vi "Speed Loop.vi"(11 "FPGA Ref":T1) -> ()   [LabVIEW 2013]
uses:
  Controls/FPGA_Reference.ctl
  Type Defs/Pump Data Mode.ctl
  <vilib>/rvi/interface/common/niFpgaWaitOnOcc.vi
  <vilib>/Utility/error.llb/Error Cluster From Error Code.vi
  <vilib>/rvi/errors/niLvFpgaAdjustHostInterfaceError.vi
  <vilib>/rvi/interface/nirviMethod/nirviMethod.xnode
  FPGA/bitfiles/TI sbRIO PWM (FPGA) v1.0.lvbitx
  <vilib>/rvi/errors/niLvFpgaMergeErrorWithErrorCode.vi
  <vilib>/FPGAPlugInAG/sbRIO-9626/niLvFpga_ReadFifo_sbRIO-9626.vi
panel:
  in  "Boolean":bool
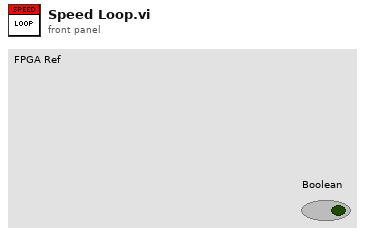
[diagram p1: front panel]
types:
  T1 = typedef "FPGA_Reference.ctl" = refnum<k20>
  T2 = cluster{"Calc 1":bool, "Calc 2":bool, "Calc 3":bool, "Calc 4":bool, "Calc 5":bool, "Calc 6":bool}
  T3 = cluster{"Array 1":dbl[], "Array 2":dbl[], "Array 3":dbl[], "Array 4":dbl[], "Array 5":dbl[], "Array 6":dbl[], "PreRead Pts":i32, "Calc Speed":cluster{"Calc 1":bool, "Calc 2":bool, "Calc 3":bool, "Calc 4":bool, "Calc 5":bool, "Calc 6":bool}, "LoopStartTime":dbl, "Speeds":dbl[], "Array 7":dbl[], "Array 8":dbl[], "Array 9":dbl[], "Array 10":dbl[], "Array 11":dbl[], "Array 12":dbl[], "Speeds 2":dbl[]}
  T4 = typedef "Pump Data Mode.ctl" = enum16{"Read", "Write Data", "Write Cal", "Write Watlow Data", "Write Pressure Offsets", "Write Initial Times", "Write Pumps Present", "Diagnostic Status", "Write Speed"}
  T5 = cluster{"max window":dbl, "min window":dbl, "CommSegments":dbl}
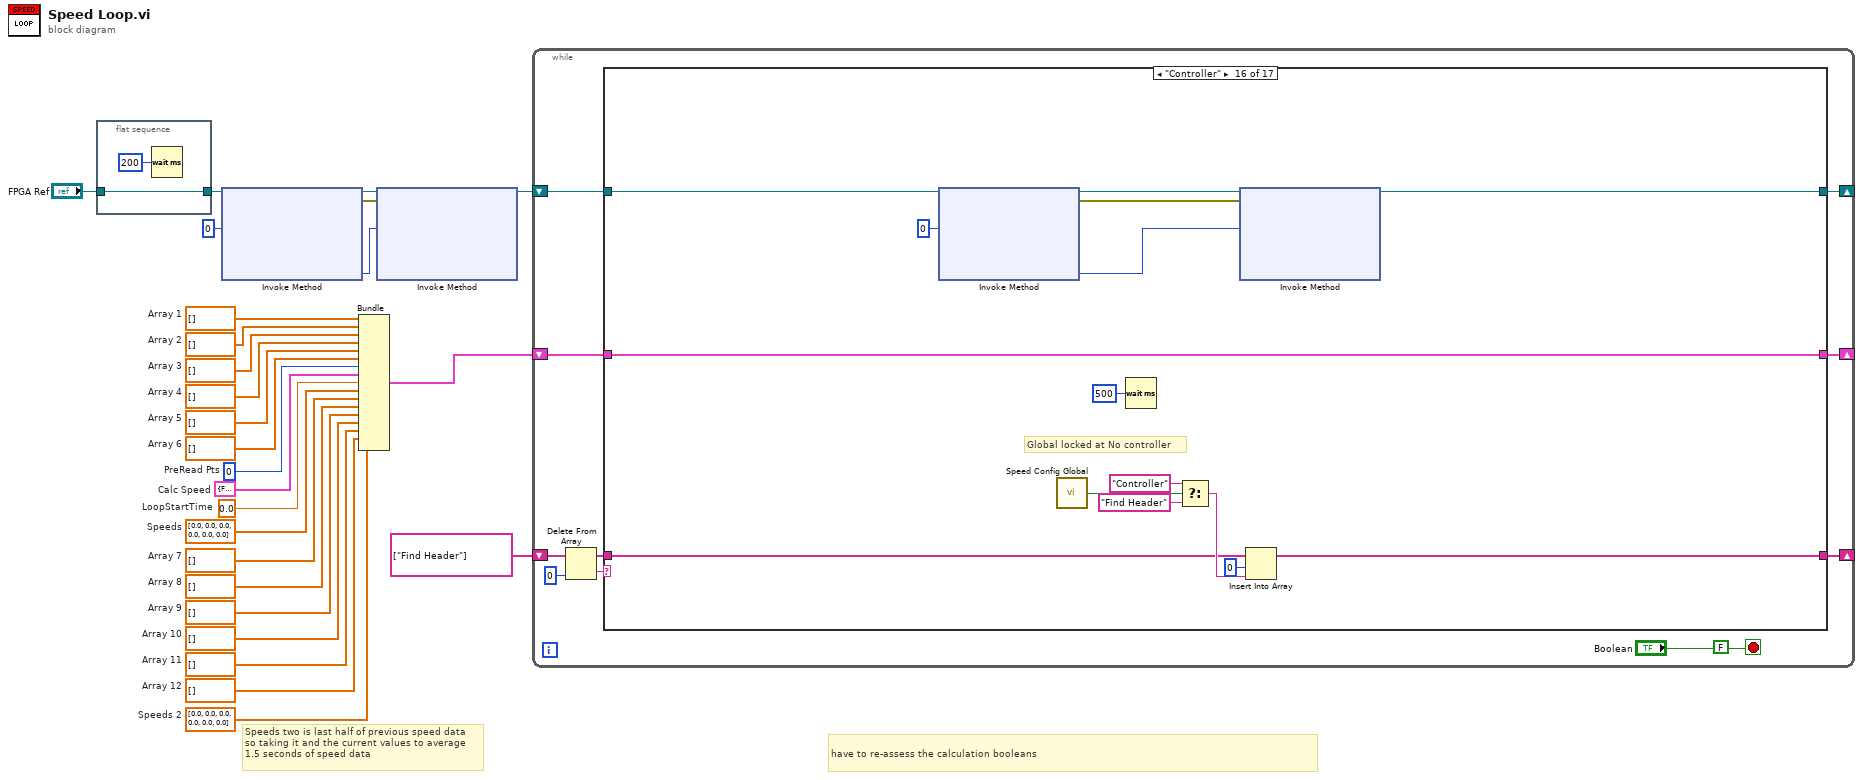
[diagram p0: block diagram]
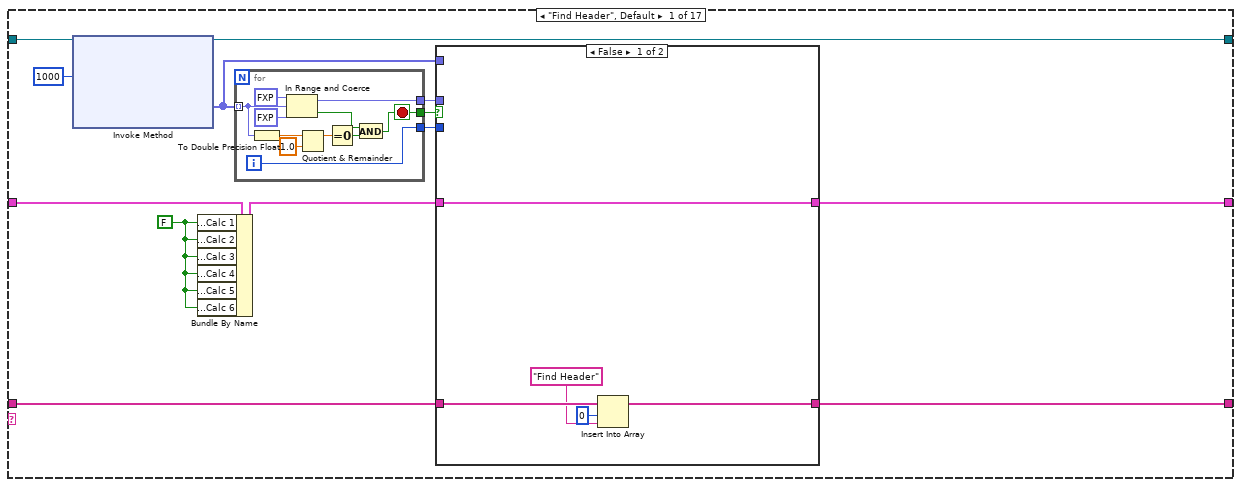
[diagram p2: hidden frame]
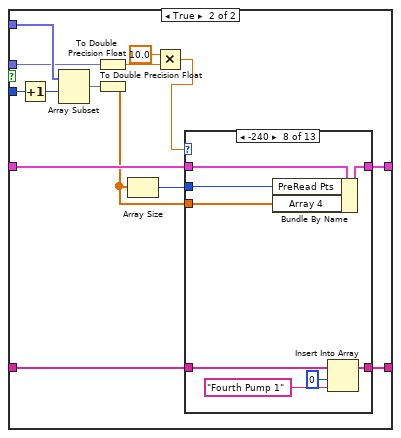
[diagram p3: hidden frame]
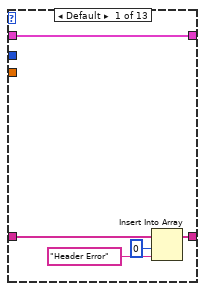
[diagram p4: hidden frame]
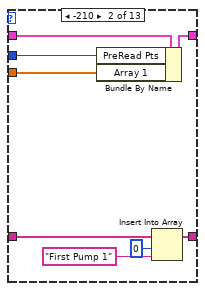
[diagram p5: hidden frame]
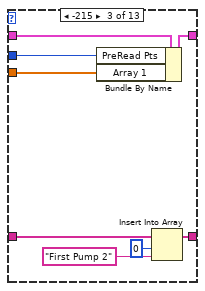
[diagram p6: hidden frame]
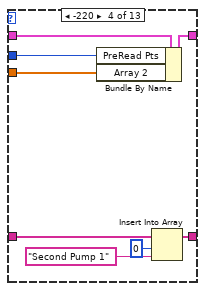
[diagram p7: hidden frame]
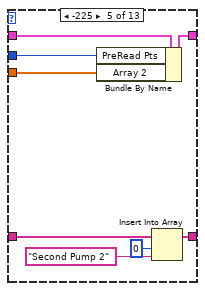
[diagram p8: hidden frame]
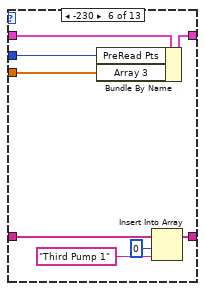
[diagram p9: hidden frame]
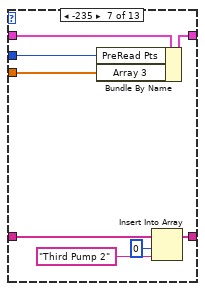
[diagram p10: hidden frame]
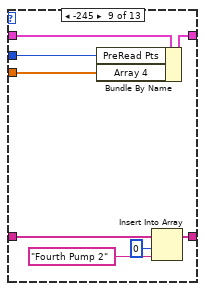
[diagram p11: hidden frame]
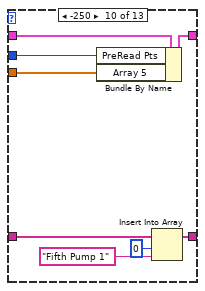
[diagram p12: hidden frame]
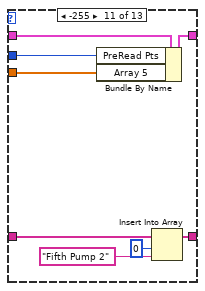
[diagram p13: hidden frame]
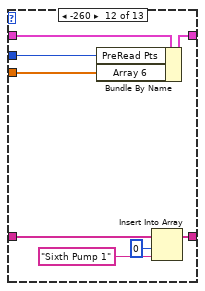
[diagram p14: hidden frame]
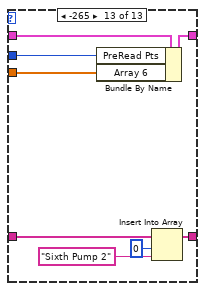
[diagram p15: hidden frame]
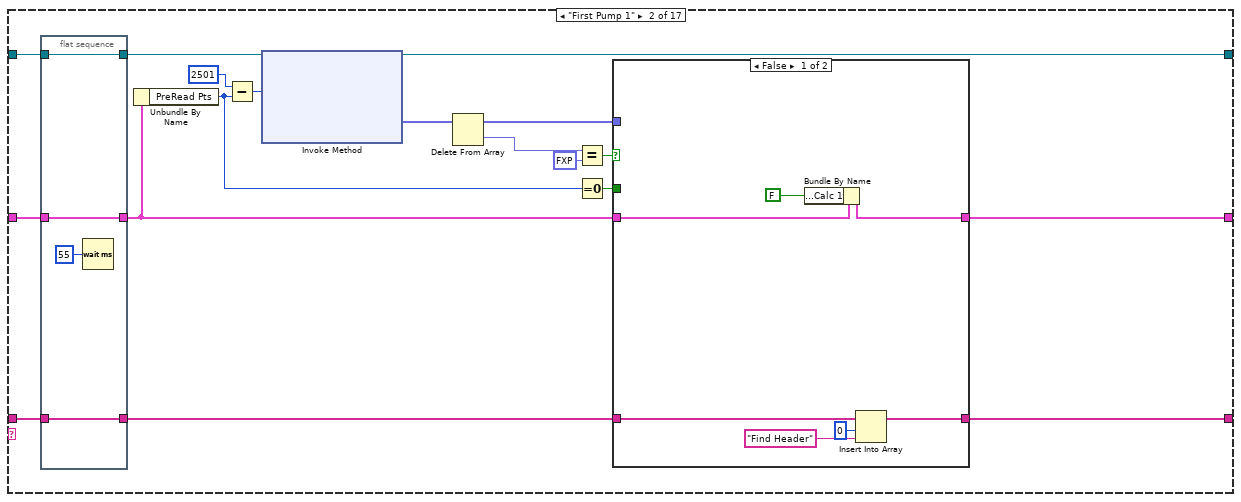
[diagram p16: hidden frame]
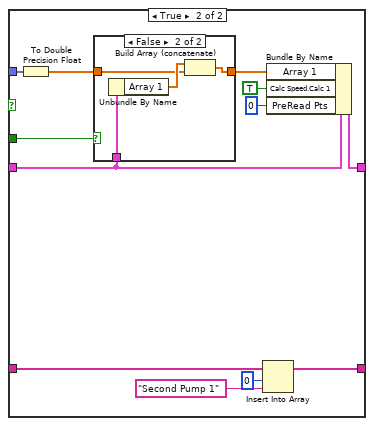
[diagram p17: hidden frame]
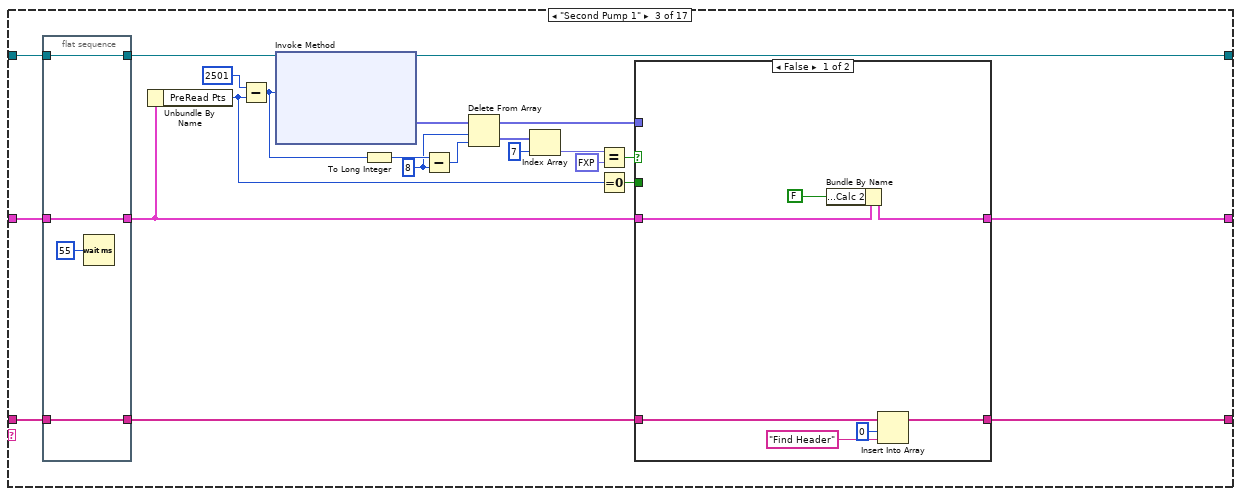
[diagram p19: hidden frame]
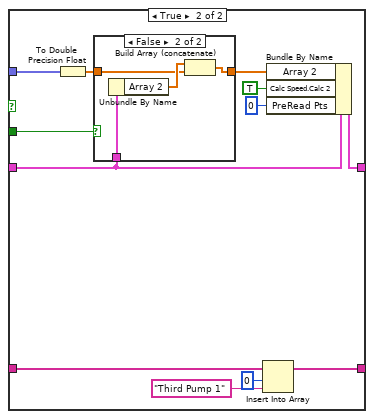
[diagram p20: hidden frame]
diagram:
  w1 = dbl[] [0.0, 0.0, 0.0, 0.0, 0.0, 0.0]  # Speeds 2
  w2 = dbl[] []  # Array 12
  w3 = dbl[] []  # Array 11
  w4 = dbl[] []  # Array 10
  w5 = dbl[] []  # Array 9
  w6 = dbl[] []  # Array 8
  w7 = dbl[] []  # Array 7
  w10 = dbl[] [0.0, 0.0, 0.0, 0.0, 0.0, 0.0]  # Speeds
  w11 = 0.0  # LoopStartTime
  w26 = T2 {"Calc 1"=FALSE, "Calc 2"=FALSE, "Calc 3"=FALSE, "Calc 4"=FALSE, "Calc 5"=FALSE, "Calc 6"=FALSE}  # Calc Speed
  w23 = 0  # PreRead Pts
  w21 = dbl[] []  # Array 6
  w20 = dbl[] []  # Array 5
  w19 = dbl[] []  # Array 4
  w18 = dbl[] []  # Array 3
  w17 = dbl[] []  # Array 2
  w16 = dbl[] []  # Array 1
  # "Speeds two is last half of previous speed data\nso taking it and the current values to average\n1.5 seconds of speed data"
  # "have to re-assess the calculation booleans"
  n1 = flat-sequence {
    tunnel: "FPGA Ref" -> [w28]
    tunnel: [w28] -> w8
    frame #0 {
      n2 = Wait (ms)(milliseconds to wait=u32 200) -> ()  [unwired: 1 out]
    }
  }
  n3 = xnode "Invoke Method"("FPGA VI Reference In"=w8, "Number of Elements"=u32 0) -> ("FPGA VI Reference Out"=w25:T1, "error out"=w13:errorcluster, "Elements Remaining"=w14:u32)  [unwired: 2 in, 1 out]
  n4 = Bundle("Array 1"=w16, "Array 2"=w17, "Array 3"=w18, "Array 4"=w19, "Array 5"=w20, "Array 6"=w21, "PreRead Pts"=w23, "Calc Speed"=w26, "LoopStartTime"=w11, "Speeds"=w10, "Array 7"=w7, "Array 8"=w6, "Array 9"=w5, "Array 10"=w4, "Array 11"=w3, "Array 12"=w2, "Speeds 2"=w1) -> (w12:T3)  [unwired: 1 in]
  n5 = xnode "Invoke Method"("FPGA VI Reference In"=w25, "error in"=w13, "Number of Elements"=w14) -> ("FPGA VI Reference Out"=w22:T1)  [unwired: 1 in, 3 out]
  n6 = while {
    shift-right: [w31] -> _
    shift-left: w22 -> [w30]
    shift-right: [w32] -> _
    shift-left: string[] ["Find Header"] -> [w38]
    shift-right: [w33] -> _
    shift-left: w12 -> [w34]
    stop <- "Boolean" stop-if-true
    (unwired) FALSE
    n7 = Delete From Array(array=w38, index=0) -> (deleted portion=w35:string, array with subset deleted=w36:string[])  [unwired: 1 in]
    n8 = case shown="\"Controller\"" w35 {
      tunnel: w30 -> [w51 w188 w240 w286 w332 w378 w424 w469 w521 w567 w613 w659 w705 w755 w860 w923 w928]
      tunnel: w34 -> [w41 w190 w242 w288 w333 w380 w426 w471 w523 w569 w614 w661 w707 w757 w859 w917 w927]
      tunnel: w36 -> [w45 w189 w241 w287 w334 w379 w425 w470 w522 w568 w615 w660 w706 w756 w858 w910 _]
      tunnel: [w44 w197 w248 w294 w340 w386 w432 w478 w529 w575 w621 w667 w713 w754 w855 w911 string[] ["Header Error"]] -> w32
      tunnel: [w43 w196 w247 w293 w339 w385 w431 w477 w528 w574 w620 w666 w712 w745 w856 w917 w927] -> w33
      tunnel: [w42 w200 w251 w297 w343 w389 w435 w481 w532 w578 w624 w670 w716 w755 w857 w918 w928] -> w31
      frame "Find Header", Default {
        w39 = FALSE ("Calc Speed.Calc 1")
        n9 = xnode "Invoke Method"("FPGA VI Reference In"=w51, "Number of Elements"=u32 1000) -> ("FPGA VI Reference Out"=w42:T1, "Data"=w46:fxp<+/-,25,6>[])  [unwired: 2 in, 2 out]
        n10 = Bundle By Name(cluster=w41, "Calc Speed.Calc 1"=w39, "Calc Speed.Calc 2"=w39, "Calc Speed.Calc 3"=w39, "Calc Speed.Calc 4"=w39, "Calc Speed.Calc 5"=w39, "Calc Speed.Calc 6"=w39) -> (w40:T3)
        n11 = for {
          tunnel: w46 -> [w178] mode=indexing
          tunnel: [w180] -> w48
          tunnel: [w172] -> w49
          tunnel: [w179] -> w47
          i -> [w179]
          stop <- w172 stop-if-true
          n12 = To Double Precision Float(number=w178) -> (double precision float=w177:dbl)
          n13 = In Range and Coerce(upper limit=fxp<+/-,25,6> -20.0, x=w178, lower limit=fxp<+/-,25,6> -27.0) -> (coerced(x)=w180:fxp<+/-,25,6>, In Range?=w173:bool)
          n14 = Quotient & Remainder(x=w177, y=1.0) -> (x-y*floor(x/y)=w175:dbl)  [unwired: 1 out]
          n15 = Equal To 0?(x=w175) -> (x = 0?=w174:bool)
          n16 = And(x=w173, y=w174) -> (x .and. y?=w172:bool)
        }
        n17 = case shown="False" w49 {
          tunnel: w48 -> [_ w60]
          tunnel: w47 -> [_ w69]
          tunnel: w46 -> [_ w70]
          tunnel: w45 -> [w56 w67]
          tunnel: [w55 w66] -> w44
          tunnel: w40 -> [w52 w65]
          tunnel: [w52 w64] -> w43
          frame False {
            n18 = Insert Into Array(array=w56, index=0, new element="Find Header") -> (w55:string[])
          }
          frame True {
            n19 = Increment(x=w69) -> (x+1=w68:i32)
            n20 = Array Subset(array=w70, index=w68) -> (w63:fxp<+/-,25,6>[])  [unwired: 1 in]
            n21 = To Double Precision Float(number=w60) -> (double precision float=w59:dbl)
            n22 = To Double Precision Float(number=w63) -> (double precision float=w62:dbl[])
            n23 = Array Size(array=w62) -> (size(s)=w61:i32)
            n24 = Multiply(x=10.0, y=w59) -> (x*y=w57:dbl)
            n25 = case shown="-240" w57 {
              tunnel: w67 -> [w73 w81 w89 w97 w105 w113 w121 w129 w137 w145 w153 w161 w169]
              tunnel: [w72 w80 w88 w96 w104 w112 w120 w128 w136 w144 w152 w160 w168] -> w66
              tunnel: w65 -> [w71 w79 w87 w95 w103 w111 w119 w127 w135 w143 w151 w159 w167]
              tunnel: [w71 w78 w86 w94 w102 w110 w118 w126 w134 w142 w150 w158 w166] -> w64
              tunnel: w62 -> [_ w77 w85 w93 w101 w109 w117 w125 w133 w141 w149 w157 w165]
              tunnel: w61 -> [_ w76 w84 w92 w100 w108 w116 w124 w132 w140 w148 w156 w164]
              frame Default {
                n26 = Insert Into Array(array=w73, index=0, new element="Header Error") -> (w72:string[])
              }
              frame -210 {
                n27 = Bundle By Name(cluster=w79, "PreRead Pts"=w76, "Array 1"=w77) -> (w78:T3)
                n28 = Insert Into Array(array=w81, index=0, new element="First Pump 1") -> (w80:string[])
              }
              frame -215 {
                n29 = Bundle By Name(cluster=w87, "PreRead Pts"=w84, "Array 1"=w85) -> (w86:T3)
                n30 = Insert Into Array(array=w89, index=0, new element="First Pump 2") -> (w88:string[])
              }
              frame -220 {
                n31 = Bundle By Name(cluster=w95, "PreRead Pts"=w92, "Array 2"=w93) -> (w94:T3)
                n32 = Insert Into Array(array=w97, index=0, new element="Second Pump 1") -> (w96:string[])
              }
              frame -225 {
                n33 = Bundle By Name(cluster=w103, "PreRead Pts"=w100, "Array 2"=w101) -> (w102:T3)
                n34 = Insert Into Array(array=w105, index=0, new element="Second Pump 2") -> (w104:string[])
              }
              frame -230 {
                n35 = Bundle By Name(cluster=w111, "PreRead Pts"=w108, "Array 3"=w109) -> (w110:T3)
                n36 = Insert Into Array(array=w113, index=0, new element="Third Pump 1") -> (w112:string[])
              }
              frame -235 {
                n37 = Bundle By Name(cluster=w119, "PreRead Pts"=w116, "Array 3"=w117) -> (w118:T3)
                n38 = Insert Into Array(array=w121, index=0, new element="Third Pump 2") -> (w120:string[])
              }
              frame -240 {
                n39 = Bundle By Name(cluster=w127, "PreRead Pts"=w124, "Array 4"=w125) -> (w126:T3)
                n40 = Insert Into Array(array=w129, index=0, new element="Fourth Pump 1") -> (w128:string[])
              }
              frame -245 {
                n41 = Bundle By Name(cluster=w135, "PreRead Pts"=w132, "Array 4"=w133) -> (w134:T3)
                n42 = Insert Into Array(array=w137, index=0, new element="Fourth Pump 2") -> (w136:string[])
              }
              frame -250 {
                n43 = Bundle By Name(cluster=w143, "PreRead Pts"=w140, "Array 5"=w141) -> (w142:T3)
                n44 = Insert Into Array(array=w145, index=0, new element="Fifth Pump 1") -> (w144:string[])
              }
              frame -255 {
                n45 = Bundle By Name(cluster=w151, "PreRead Pts"=w148, "Array 5"=w149) -> (w150:T3)
                n46 = Insert Into Array(array=w153, index=0, new element="Fifth Pump 2") -> (w152:string[])
              }
              frame -260 {
                n47 = Bundle By Name(cluster=w159, "PreRead Pts"=w156, "Array 6"=w157) -> (w158:T3)
                n48 = Insert Into Array(array=w161, index=0, new element="Sixth Pump 1") -> (w160:string[])
              }
              frame -265 {
                n49 = Bundle By Name(cluster=w167, "PreRead Pts"=w164, "Array 6"=w165) -> (w166:T3)
                n50 = Insert Into Array(array=w169, index=0, new element="Sixth Pump 2") -> (w168:string[])
              }
            }
          }
        }
      }
      frame "First Pump 1" {
        n51 = flat-sequence {
          tunnel: w190 -> [w202]
          tunnel: w189 -> [w203]
          tunnel: w188 -> [w201]
          tunnel: [w203] -> w187
          tunnel: [w202] -> w186
          tunnel: [w201] -> w185
          frame #0 {
            n52 = Wait (ms)(milliseconds to wait=u32 55) -> ()  [unwired: 1 out]
          }
        }
        n53 = Unbundle By Name(w186) -> ("PreRead Pts"=w192:i32)
        n54 = Subtract(x=u32 2501 ("Number of Elements"), y=w192) -> (x-y=w184:u32)
        n55 = xnode "Invoke Method"("FPGA VI Reference In"=w185, "Number of Elements"=w184) -> ("FPGA VI Reference Out"=w200:T1, "Data"=w198:fxp<+/-,25,6>[])  [unwired: 2 in, 2 out]
        n56 = Delete From Array(array=w198) -> (deleted portion=w183:fxp<+/-,25,6>, array with subset deleted=w195:fxp<+/-,25,6>[])  [unwired: 2 in]
        n57 = Equal?(x=w183, y=fxp<+/-,25,6> -22.0 ("lower limit")) -> (x = y?=w193:bool)
        n58 = Equal To 0?(x=w192) -> (x = 0?=w191:bool)
        n59 = case shown="False" w193 {
          tunnel: w186 -> [w208 w222]
          tunnel: w187 -> [w206 w215]
          tunnel: [w205 w214] -> w197
          tunnel: [w207 w223] -> w196
          tunnel: w195 -> [_ w220]
          tunnel: w191 -> [_ w221]
          frame False {
            n60 = Bundle By Name(cluster=w208, "Calc Speed.Calc 1"=FALSE) -> (w207:T3)
            n61 = Insert Into Array(array=w206, index=0, new element="Find Header") -> (w205:string[])
          }
          frame True {
            n62 = To Double Precision Float(number=w220) -> (double precision float=w219:dbl[])
            n63 = case shown="False" w221 {
              tunnel: w222 -> [_ w228]
              tunnel: w219 -> [w224 w226]
              tunnel: [w224 w225] -> w218
              frame True {
              }
              frame False {
                n64 = Unbundle By Name(w228) -> ("Array 1"=w227:dbl[])
                n65 = Build Array (concatenate)(w227, w226) -> (w225:dbl[])
              }
            }
            n66 = Insert Into Array(array=w215, index=0, new element="Second Pump 1") -> (w214:string[])
            n67 = Bundle By Name(cluster=w222, "Array 1"=w218, "Calc Speed.Calc 1"=TRUE, "PreRead Pts"=0) -> (w223:T3)
          }
        }
      }
      frame "Second Pump 1" {
        w232 = 8 ("length")
        n68 = flat-sequence {
          tunnel: w242 -> [w253]
          tunnel: w241 -> [w254]
          tunnel: w240 -> [w252]
          tunnel: [w254] -> w239
          tunnel: [w253] -> w238
          tunnel: [w252] -> w237
          frame #0 {
            n69 = Wait (ms)(milliseconds to wait=u32 55) -> ()  [unwired: 1 out]
          }
        }
        n70 = Unbundle By Name(w238) -> ("PreRead Pts"=w231:i32)
        n71 = Subtract(x=u32 2501 ("Number of Elements"), y=w231) -> (x-y=w229:u32)
        n72 = xnode "Invoke Method"("FPGA VI Reference In"=w237, "Number of Elements"=w229) -> ("FPGA VI Reference Out"=w251:T1, "Data"=w249:fxp<+/-,25,6>[])  [unwired: 2 in, 2 out]
        n73 = To Long Integer(number=w229) -> (32bit integer=w233:i32)
        n74 = Subtract(x=w233, y=w232) -> (x-y=w230:i32)
        n75 = Delete From Array(array=w249, length=w232, index=w230) -> (deleted portion=w236:fxp<+/-,25,6>[], array with subset deleted=w246:fxp<+/-,25,6>[])
        n76 = Index Array(array=w236, index=7) -> (element=w234:fxp<+/-,25,6>)
        n77 = Equal?(x=w234, y=fxp<+/-,25,6> -23.0 ("lower limit")) -> (x = y?=w244:bool)
        n78 = Equal To 0?(x=w231) -> (x = 0?=w243:bool)
        n79 = case shown="False" w244 {
          tunnel: w238 -> [w259 w273]
          tunnel: w239 -> [w257 w266]
          tunnel: [w256 w265] -> w248
          tunnel: [w258 w274] -> w247
          tunnel: w246 -> [_ w271]
          tunnel: w243 -> [_ w272]
          frame False {
            n80 = Bundle By Name(cluster=w259, "Calc Speed.Calc 2"=FALSE ("Calc Speed.Calc 1")) -> (w258:T3)
            n81 = Insert Into Array(array=w257, index=0, new element="Find Header") -> (w256:string[])
          }
          frame True {
            n82 = To Double Precision Float(number=w271) -> (double precision float=w270:dbl[])
            n83 = case shown="False" w272 {
              tunnel: w273 -> [_ w279]
              tunnel: w270 -> [w275 w277]
              tunnel: [w275 w276] -> w269
              frame True {
              }
              frame False {
                n84 = Unbundle By Name(w279) -> ("Array 2"=w278:dbl[])
                n85 = Build Array (concatenate)(w278, w277) -> (w276:dbl[])
              }
            }
            n86 = Insert Into Array(array=w266, index=0, new element="Third Pump 1") -> (w265:string[])
            n87 = Bundle By Name(cluster=w273, "Array 2"=w269, "Calc Speed.Calc 2"=TRUE ("Calc Speed.Calc 1"), "PreRead Pts"=0) -> (w274:T3)
          }
        }
      }
      frame "Third Pump 1" {
        n88 = flat-sequence {
          tunnel: w288 -> [w299]
          tunnel: w287 -> [w300]
          tunnel: w286 -> [w298]
          tunnel: [w300] -> w285
          tunnel: [w299] -> w284
          tunnel: [w298] -> w283
          frame #0 {
            n89 = Wait (ms)(milliseconds to wait=u32 55) -> ()  [unwired: 1 out]
          }
        }
        n90 = Unbundle By Name(w284) -> ("PreRead Pts"=w282:i32)
        n91 = Subtract(x=u32 2501 ("Number of Elements"), y=w282) -> (x-y=w281:u32)
        n92 = xnode "Invoke Method"("FPGA VI Reference In"=w283, "Number of Elements"=w281) -> ("FPGA VI Reference Out"=w297:T1, "Data"=w295:fxp<+/-,25,6>[])  [unwired: 2 in, 2 out]
        n93 = Delete From Array(array=w295) -> (deleted portion=w280:fxp<+/-,25,6>, array with subset deleted=w292:fxp<+/-,25,6>[])  [unwired: 2 in]
        n94 = Equal?(x=w280, y=fxp<+/-,25,6> -24.0 ("lower limit")) -> (x = y?=w290:bool)
        n95 = Equal To 0?(x=w282) -> (x = 0?=w289:bool)
        n96 = case shown="False" w290 {
          tunnel: w284 -> [w305 w319]
          tunnel: w285 -> [w303 w312]
          tunnel: [w302 w311] -> w294
          tunnel: [w304 w320] -> w293
          tunnel: w292 -> [_ w317]
          tunnel: w289 -> [_ w318]
          frame False {
            n97 = Bundle By Name(cluster=w305, "Calc Speed.Calc 3"=FALSE ("Calc Speed.Calc 1")) -> (w304:T3)
            n98 = Insert Into Array(array=w303, index=0, new element="Find Header") -> (w302:string[])
          }
          frame True {
            n99 = To Double Precision Float(number=w317) -> (double precision float=w316:dbl[])
            n100 = case shown="False" w318 {
              tunnel: w319 -> [_ w325]
              tunnel: w316 -> [w321 w323]
              tunnel: [w321 w322] -> w315
              frame True {
              }
              frame False {
                n101 = Unbundle By Name(w325) -> ("Array 3"=w324:dbl[])
                n102 = Build Array (concatenate)(w324, w323) -> (w322:dbl[])
              }
            }
            n103 = Insert Into Array(array=w312, index=0, new element="Fourth Pump 1") -> (w311:string[])
            n104 = Bundle By Name(cluster=w319, "Array 3"=w315, "Calc Speed.Calc 3"=TRUE ("Calc Speed.Calc 1"), "PreRead Pts"=0) -> (w320:T3)
          }
        }
      }
      frame "Fourth Pump 1" {
        n105 = flat-sequence {
          tunnel: w334 -> [w346]
          tunnel: w333 -> [w345]
          tunnel: w332 -> [w344]
          tunnel: [w346] -> w331
          tunnel: [w345] -> w330
          tunnel: [w344] -> w329
          frame #0 {
            n106 = Wait (ms)(milliseconds to wait=u32 55) -> ()  [unwired: 1 out]
          }
        }
        n107 = Unbundle By Name(w330) -> ("PreRead Pts"=w328:i32)
        n108 = Subtract(x=u32 2501 ("Number of Elements"), y=w328) -> (x-y=w327:u32)
        n109 = xnode "Invoke Method"("FPGA VI Reference In"=w329, "Number of Elements"=w327) -> ("FPGA VI Reference Out"=w343:T1, "Data"=w341:fxp<+/-,25,6>[])  [unwired: 2 in, 2 out]
        n110 = Delete From Array(array=w341) -> (deleted portion=w326:fxp<+/-,25,6>, array with subset deleted=w338:fxp<+/-,25,6>[])  [unwired: 2 in]
        n111 = Equal?(x=w326, y=fxp<+/-,25,6> -25.0 ("lower limit")) -> (x = y?=w336:bool)
        n112 = Equal To 0?(x=w328) -> (x = 0?=w335:bool)
        n113 = case shown="True" w336 {
          tunnel: w330 -> [w351 w365]
          tunnel: w331 -> [w349 w358]
          tunnel: [w348 w357] -> w340
          tunnel: [w350 w366] -> w339
          tunnel: w338 -> [_ w363]
          tunnel: w335 -> [_ w364]
          frame False {
            n114 = Bundle By Name(cluster=w351, "Calc Speed.Calc 4"=FALSE ("Calc Speed.Calc 1")) -> (w350:T3)
            n115 = Insert Into Array(array=w349, index=0, new element="Find Header") -> (w348:string[])
          }
          frame True {
            n116 = To Double Precision Float(number=w363) -> (double precision float=w362:dbl[])
            n117 = case shown="False" w364 {
              tunnel: w365 -> [_ w371]
              tunnel: w362 -> [w367 w369]
              tunnel: [w367 w368] -> w361
              frame True {
              }
              frame False {
                n118 = Unbundle By Name(w371) -> ("Array 4"=w370:dbl[])
                n119 = Build Array (concatenate)(w370, w369) -> (w368:dbl[])
              }
            }
            n120 = Insert Into Array(array=w358, index=0, new element="Fifth Pump 1") -> (w357:string[])
            n121 = Bundle By Name(cluster=w365, "Array 4"=w361, "Calc Speed.Calc 4"=TRUE ("Calc Speed.Calc 1"), "PreRead Pts"=0) -> (w366:T3)
          }
        }
      }
      frame "Fifth Pump 1" {
        n122 = flat-sequence {
          tunnel: w380 -> [w391]
          tunnel: w379 -> [w392]
          tunnel: w378 -> [w390]
          tunnel: [w392] -> w377
          tunnel: [w391] -> w376
          tunnel: [w390] -> w375
          frame #0 {
            n123 = Wait (ms)(milliseconds to wait=u32 55) -> ()  [unwired: 1 out]
          }
        }
        n124 = Unbundle By Name(w376) -> ("PreRead Pts"=w374:i32)
        n125 = Subtract(x=u32 2501 ("Number of Elements"), y=w374) -> (x-y=w373:u32)
        n126 = xnode "Invoke Method"("FPGA VI Reference In"=w375, "Number of Elements"=w373) -> ("FPGA VI Reference Out"=w389:T1, "Data"=w387:fxp<+/-,25,6>[])  [unwired: 2 in, 2 out]
        n127 = Delete From Array(array=w387) -> (deleted portion=w372:fxp<+/-,25,6>, array with subset deleted=w384:fxp<+/-,25,6>[])  [unwired: 2 in]
        n128 = Equal?(x=w372, y=fxp<+/-,25,6> -26.0 ("lower limit")) -> (x = y?=w382:bool)
        n129 = Equal To 0?(x=w374) -> (x = 0?=w381:bool)
        n130 = case shown="False" w382 {
          tunnel: w376 -> [w397 w411]
          tunnel: w377 -> [w395 w404]
          tunnel: [w394 w403] -> w386
          tunnel: [w396 w412] -> w385
          tunnel: w384 -> [_ w409]
          tunnel: w381 -> [_ w410]
          frame False {
            n131 = Bundle By Name(cluster=w397, "Calc Speed.Calc 5"=FALSE ("Calc Speed.Calc 1")) -> (w396:T3)
            n132 = Insert Into Array(array=w395, index=0, new element="Find Header") -> (w394:string[])
          }
          frame True {
            n133 = To Double Precision Float(number=w409) -> (double precision float=w408:dbl[])
            n134 = case shown="False" w410 {
              tunnel: w411 -> [_ w417]
              tunnel: w408 -> [w413 w415]
              tunnel: [w413 w414] -> w407
              frame True {
              }
              frame False {
                n135 = Unbundle By Name(w417) -> ("Array 5"=w416:dbl[])
                n136 = Build Array (concatenate)(w416, w415) -> (w414:dbl[])
              }
            }
            n137 = Insert Into Array(array=w404, index=0, new element="Sixth Pump 1") -> (w403:string[])
            n138 = Bundle By Name(cluster=w411, "Array 5"=w407, "Calc Speed.Calc 5"=TRUE ("Calc Speed.Calc 1"), "PreRead Pts"=0) -> (w412:T3)
          }
        }
      }
      frame "Sixth Pump 1" {
        n139 = flat-sequence {
          tunnel: w426 -> [w437]
          tunnel: w425 -> [w438]
          tunnel: w424 -> [w436]
          tunnel: [w438] -> w423
          tunnel: [w437] -> w422
          tunnel: [w436] -> w421
          frame #0 {
            n140 = Wait (ms)(milliseconds to wait=u32 55) -> ()  [unwired: 1 out]
          }
        }
        n141 = Unbundle By Name(w422) -> ("PreRead Pts"=w420:i32)
        n142 = Subtract(x=u32 2501 ("Number of Elements"), y=w420) -> (x-y=w419:u32)
        n143 = xnode "Invoke Method"("FPGA VI Reference In"=w421, "Number of Elements"=w419) -> ("FPGA VI Reference Out"=w435:T1, "Data"=w433:fxp<+/-,25,6>[])  [unwired: 2 in, 2 out]
        n144 = Delete From Array(array=w433) -> (deleted portion=w418:fxp<+/-,25,6>, array with subset deleted=w430:fxp<+/-,25,6>[])  [unwired: 2 in]
        n145 = Equal?(x=w418, y=fxp<+/-,25,6> -21.5 ("lower limit")) -> (x = y?=w428:bool)
        n146 = Equal To 0?(x=w420) -> (x = 0?=w427:bool)
        n147 = case shown="False" w428 {
          tunnel: w422 -> [w443 w457]
          tunnel: w423 -> [w441 w450]
          tunnel: [w440 w449] -> w432
          tunnel: [w442 w458] -> w431
          tunnel: w430 -> [_ w455]
          tunnel: w427 -> [_ w456]
          frame False {
            n148 = Bundle By Name(cluster=w443, "Calc Speed.Calc 6"=FALSE ("Calc Speed.Calc 1")) -> (w442:T3)
            n149 = Insert Into Array(array=w441, index=0, new element="Find Header") -> (w440:string[])
          }
          frame True {
            n150 = To Double Precision Float(number=w455) -> (double precision float=w454:dbl[])
            n151 = case shown="False" w456 {
              tunnel: w457 -> [_ w463]
              tunnel: w454 -> [w459 w461]
              tunnel: [w459 w460] -> w453
              frame True {
              }
              frame False {
                n152 = Unbundle By Name(w463) -> ("Array 6"=w462:dbl[])
                n153 = Build Array (concatenate)(w462, w461) -> (w460:dbl[])
              }
            }
            n154 = Insert Into Array(array=w450, index=0, new element="First Pump 2") -> (w449:string[])
            n155 = Bundle By Name(cluster=w457, "Array 6"=w453, "Calc Speed.Calc 6"=TRUE ("Calc Speed.Calc 1"), "PreRead Pts"=0) -> (w458:T3)
          }
        }
      }
      frame "First Pump 2" {
        n156 = flat-sequence {
          tunnel: w471 -> [w483]
          tunnel: w470 -> [w484]
          tunnel: w469 -> [w482]
          tunnel: [w484] -> w468
          tunnel: [w483] -> w467
          tunnel: [w482] -> w466
          frame #0 {
            n157 = Wait (ms)(milliseconds to wait=u32 55) -> ()  [unwired: 1 out]
          }
        }
        n158 = Unbundle By Name(w467) -> ("PreRead Pts"=w473:i32)
        n159 = Subtract(x=u32 2501 ("Number of Elements"), y=w473) -> (x-y=w465:u32)
        n160 = xnode "Invoke Method"("FPGA VI Reference In"=w466, "Number of Elements"=w465) -> ("FPGA VI Reference Out"=w481:T1, "Data"=w479:fxp<+/-,25,6>[])  [unwired: 2 in, 2 out]
        n161 = Delete From Array(array=w479) -> (deleted portion=w464:fxp<+/-,25,6>, array with subset deleted=w476:fxp<+/-,25,6>[])  [unwired: 2 in]
        n162 = Equal?(x=w464, y=fxp<+/-,25,6> -22.5 ("lower limit")) -> (x = y?=w474:bool)
        n163 = Equal To 0?(x=w473) -> (x = 0?=w472:bool)
        n164 = case shown="False" w474 {
          tunnel: w467 -> [w489 w503]
          tunnel: w468 -> [w487 w496]
          tunnel: [w486 w495] -> w478
          tunnel: [w488 w504] -> w477
          tunnel: w476 -> [_ w501]
          tunnel: w472 -> [_ w502]
          frame False {
            n165 = Bundle By Name(cluster=w489, "Calc Speed.Calc 1"=FALSE) -> (w488:T3)
            n166 = Insert Into Array(array=w487, index=0, new element="Find Header") -> (w486:string[])
          }
          frame True {
            n167 = To Double Precision Float(number=w501) -> (double precision float=w500:dbl[])
            n168 = case shown="False" w502 {
              tunnel: w503 -> [_ w509]
              tunnel: w500 -> [w505 w507]
              tunnel: [w505 w506] -> w499
              frame True {
              }
              frame False {
                n169 = Unbundle By Name(w509) -> ("Array 7"=w508:dbl[])
                n170 = Build Array (concatenate)(w508, w507) -> (w506:dbl[])
              }
            }
            n171 = Insert Into Array(array=w496, index=0, new element="Second Pump 2") -> (w495:string[])
            n172 = Bundle By Name(cluster=w503, "Array 7"=w499, "Calc Speed.Calc 1"=TRUE, "PreRead Pts"=0) -> (w504:T3)
          }
        }
      }
      frame "Second Pump 2" {
        w513 = 8 ("length")
        n173 = flat-sequence {
          tunnel: w523 -> [w534]
          tunnel: w522 -> [w535]
          tunnel: w521 -> [w533]
          tunnel: [w535] -> w520
          tunnel: [w534] -> w519
          tunnel: [w533] -> w518
          frame #0 {
            n174 = Wait (ms)(milliseconds to wait=u32 55) -> ()  [unwired: 1 out]
          }
        }
        n175 = Unbundle By Name(w519) -> ("PreRead Pts"=w512:i32)
        n176 = Subtract(x=u32 2501 ("Number of Elements"), y=w512) -> (x-y=w510:u32)
        n177 = xnode "Invoke Method"("FPGA VI Reference In"=w518, "Number of Elements"=w510) -> ("FPGA VI Reference Out"=w532:T1, "Data"=w530:fxp<+/-,25,6>[])  [unwired: 2 in, 2 out]
        n178 = To Long Integer(number=w510) -> (32bit integer=w514:i32)
        n179 = Subtract(x=w514, y=w513) -> (x-y=w511:i32)
        n180 = Delete From Array(array=w530, length=w513, index=w511) -> (deleted portion=w517:fxp<+/-,25,6>[], array with subset deleted=w527:fxp<+/-,25,6>[])
        n181 = Index Array(array=w517, index=7) -> (element=w515:fxp<+/-,25,6>)
        n182 = Equal?(x=w515, y=fxp<+/-,25,6> -23.5 ("lower limit")) -> (x = y?=w525:bool)
        n183 = Equal To 0?(x=w512) -> (x = 0?=w524:bool)
        n184 = case shown="False" w525 {
          tunnel: w519 -> [w540 w554]
          tunnel: w520 -> [w538 w547]
          tunnel: [w537 w546] -> w529
          tunnel: [w539 w555] -> w528
          tunnel: w527 -> [_ w552]
          tunnel: w524 -> [_ w553]
          frame False {
            n185 = Bundle By Name(cluster=w540, "Calc Speed.Calc 2"=FALSE ("Calc Speed.Calc 1")) -> (w539:T3)
            n186 = Insert Into Array(array=w538, index=0, new element="Find Header") -> (w537:string[])
          }
          frame True {
            n187 = To Double Precision Float(number=w552) -> (double precision float=w551:dbl[])
            n188 = case shown="False" w553 {
              tunnel: w554 -> [_ w560]
              tunnel: w551 -> [w556 w558]
              tunnel: [w556 w557] -> w550
              frame True {
              }
              frame False {
                n189 = Unbundle By Name(w560) -> ("Array 8"=w559:dbl[])
                n190 = Build Array (concatenate)(w559, w558) -> (w557:dbl[])
              }
            }
            n191 = Insert Into Array(array=w547, index=0, new element="Third Pump 2") -> (w546:string[])
            n192 = Bundle By Name(cluster=w554, "Array 8"=w550, "Calc Speed.Calc 2"=TRUE ("Calc Speed.Calc 1"), "PreRead Pts"=0) -> (w555:T3)
          }
        }
      }
      frame "Third Pump 2" {
        n193 = flat-sequence {
          tunnel: w569 -> [w580]
          tunnel: w568 -> [w581]
          tunnel: w567 -> [w579]
          tunnel: [w581] -> w566
          tunnel: [w580] -> w565
          tunnel: [w579] -> w564
          frame #0 {
            n194 = Wait (ms)(milliseconds to wait=u32 55) -> ()  [unwired: 1 out]
          }
        }
        n195 = Unbundle By Name(w565) -> ("PreRead Pts"=w563:i32)
        n196 = Subtract(x=u32 2501 ("Number of Elements"), y=w563) -> (x-y=w562:u32)
        n197 = xnode "Invoke Method"("FPGA VI Reference In"=w564, "Number of Elements"=w562) -> ("FPGA VI Reference Out"=w578:T1, "Data"=w576:fxp<+/-,25,6>[])  [unwired: 2 in, 2 out]
        n198 = Delete From Array(array=w576) -> (deleted portion=w561:fxp<+/-,25,6>, array with subset deleted=w573:fxp<+/-,25,6>[])  [unwired: 2 in]
        n199 = Equal?(x=w561, y=fxp<+/-,25,6> -24.5 ("lower limit")) -> (x = y?=w571:bool)
        n200 = Equal To 0?(x=w563) -> (x = 0?=w570:bool)
        n201 = case shown="True" w571 {
          tunnel: w565 -> [w586 w600]
          tunnel: w566 -> [w584 w593]
          tunnel: [w583 w592] -> w575
          tunnel: [w585 w601] -> w574
          tunnel: w573 -> [_ w598]
          tunnel: w570 -> [_ w599]
          frame False {
            n202 = Bundle By Name(cluster=w586, "Calc Speed.Calc 3"=FALSE ("Calc Speed.Calc 1")) -> (w585:T3)
            n203 = Insert Into Array(array=w584, index=0, new element="Find Header") -> (w583:string[])
          }
          frame True {
            n204 = To Double Precision Float(number=w598) -> (double precision float=w597:dbl[])
            n205 = case shown="False" w599 {
              tunnel: w600 -> [_ w606]
              tunnel: w597 -> [w602 w604]
              tunnel: [w602 w603] -> w596
              frame True {
              }
              frame False {
                n206 = Unbundle By Name(w606) -> ("Array 9"=w605:dbl[])
                n207 = Build Array (concatenate)(w605, w604) -> (w603:dbl[])
              }
            }
            n208 = Insert Into Array(array=w593, index=0, new element="Fourth Pump 2") -> (w592:string[])
            n209 = Bundle By Name(cluster=w600, "Array 9"=w596, "Calc Speed.Calc 3"=TRUE ("Calc Speed.Calc 1"), "PreRead Pts"=0) -> (w601:T3)
          }
        }
      }
      frame "Fourth Pump 2" {
        n210 = flat-sequence {
          tunnel: w615 -> [w627]
          tunnel: w614 -> [w626]
          tunnel: w613 -> [w625]
          tunnel: [w627] -> w612
          tunnel: [w626] -> w611
          tunnel: [w625] -> w610
          frame #0 {
            n211 = Wait (ms)(milliseconds to wait=u32 55) -> ()  [unwired: 1 out]
          }
        }
        n212 = Unbundle By Name(w611) -> ("PreRead Pts"=w609:i32)
        n213 = Subtract(x=u32 2501 ("Number of Elements"), y=w609) -> (x-y=w608:u32)
        n214 = xnode "Invoke Method"("FPGA VI Reference In"=w610, "Number of Elements"=w608) -> ("FPGA VI Reference Out"=w624:T1, "Data"=w622:fxp<+/-,25,6>[])  [unwired: 2 in, 2 out]
        n215 = Delete From Array(array=w622) -> (deleted portion=w607:fxp<+/-,25,6>, array with subset deleted=w619:fxp<+/-,25,6>[])  [unwired: 2 in]
        n216 = Equal?(x=w607, y=fxp<+/-,25,6> -25.5 ("lower limit")) -> (x = y?=w617:bool)
        n217 = Equal To 0?(x=w609) -> (x = 0?=w616:bool)
        n218 = case shown="False" w617 {
          tunnel: w611 -> [w632 w646]
          tunnel: w612 -> [w630 w639]
          tunnel: [w629 w638] -> w621
          tunnel: [w631 w647] -> w620
          tunnel: w619 -> [_ w644]
          tunnel: w616 -> [_ w645]
          frame False {
            n219 = Bundle By Name(cluster=w632, "Calc Speed.Calc 4"=FALSE ("Calc Speed.Calc 1")) -> (w631:T3)
            n220 = Insert Into Array(array=w630, index=0, new element="Find Header") -> (w629:string[])
          }
          frame True {
            n221 = To Double Precision Float(number=w644) -> (double precision float=w643:dbl[])
            n222 = case shown="False" w645 {
              tunnel: w646 -> [_ w652]
              tunnel: w643 -> [w648 w650]
              tunnel: [w648 w649] -> w642
              frame True {
              }
              frame False {
                n223 = Unbundle By Name(w652) -> ("Array 10"=w651:dbl[])
                n224 = Build Array (concatenate)(w651, w650) -> (w649:dbl[])
              }
            }
            n225 = Insert Into Array(array=w639, index=0, new element="Fifth Pump 2") -> (w638:string[])
            n226 = Bundle By Name(cluster=w646, "Array 10"=w642, "Calc Speed.Calc 4"=TRUE ("Calc Speed.Calc 1"), "PreRead Pts"=0) -> (w647:T3)
          }
        }
      }
      frame "Fifth Pump 2" {
        n227 = flat-sequence {
          tunnel: w661 -> [w672]
          tunnel: w660 -> [w673]
          tunnel: w659 -> [w671]
          tunnel: [w673] -> w658
          tunnel: [w672] -> w657
          tunnel: [w671] -> w656
          frame #0 {
            n228 = Wait (ms)(milliseconds to wait=u32 55) -> ()  [unwired: 1 out]
          }
        }
        n229 = Unbundle By Name(w657) -> ("PreRead Pts"=w655:i32)
        n230 = Subtract(x=u32 2501 ("Number of Elements"), y=w655) -> (x-y=w654:u32)
        n231 = xnode "Invoke Method"("FPGA VI Reference In"=w656, "Number of Elements"=w654) -> ("FPGA VI Reference Out"=w670:T1, "Data"=w668:fxp<+/-,25,6>[])  [unwired: 2 in, 2 out]
        n232 = Delete From Array(array=w668) -> (deleted portion=w653:fxp<+/-,25,6>, array with subset deleted=w665:fxp<+/-,25,6>[])  [unwired: 2 in]
        n233 = Equal?(x=w653, y=fxp<+/-,25,6> -26.5 ("lower limit")) -> (x = y?=w663:bool)
        n234 = Equal To 0?(x=w655) -> (x = 0?=w662:bool)
        n235 = case shown="False" w663 {
          tunnel: w657 -> [w678 w692]
          tunnel: w658 -> [w676 w685]
          tunnel: [w675 w684] -> w667
          tunnel: [w677 w693] -> w666
          tunnel: w665 -> [_ w690]
          tunnel: w662 -> [_ w691]
          frame False {
            n236 = Bundle By Name(cluster=w678, "Calc Speed.Calc 5"=FALSE ("Calc Speed.Calc 1")) -> (w677:T3)
            n237 = Insert Into Array(array=w676, index=0, new element="Find Header") -> (w675:string[])
          }
          frame True {
            n238 = To Double Precision Float(number=w690) -> (double precision float=w689:dbl[])
            n239 = case shown="False" w691 {
              tunnel: w692 -> [_ w698]
              tunnel: w689 -> [w694 w696]
              tunnel: [w694 w695] -> w688
              frame True {
              }
              frame False {
                n240 = Unbundle By Name(w698) -> ("Array 11"=w697:dbl[])
                n241 = Build Array (concatenate)(w697, w696) -> (w695:dbl[])
              }
            }
            n242 = Insert Into Array(array=w685, index=0, new element="Sixth Pump 2") -> (w684:string[])
            n243 = Bundle By Name(cluster=w692, "Array 11"=w688, "Calc Speed.Calc 5"=TRUE ("Calc Speed.Calc 1"), "PreRead Pts"=0) -> (w693:T3)
          }
        }
      }
      frame "Sixth Pump 2" {
        n244 = flat-sequence {
          tunnel: w707 -> [w718]
          tunnel: w706 -> [w719]
          tunnel: w705 -> [w717]
          tunnel: [w719] -> w704
          tunnel: [w718] -> w703
          tunnel: [w717] -> w702
          frame #0 {
            n245 = Wait (ms)(milliseconds to wait=u32 55) -> ()  [unwired: 1 out]
          }
        }
        n246 = Unbundle By Name(w703) -> ("PreRead Pts"=w701:i32)
        n247 = Subtract(x=u32 2501 ("Number of Elements"), y=w701) -> (x-y=w700:u32)
        n248 = xnode "Invoke Method"("FPGA VI Reference In"=w702, "Number of Elements"=w700) -> ("FPGA VI Reference Out"=w716:T1, "Data"=w714:fxp<+/-,25,6>[])  [unwired: 2 in, 2 out]
        n249 = Delete From Array(array=w714) -> (deleted portion=w699:fxp<+/-,25,6>, array with subset deleted=w711:fxp<+/-,25,6>[])  [unwired: 2 in]
        n250 = Equal?(x=w699, y=fxp<+/-,25,6> -31.0 ("lower limit")) -> (x = y?=w709:bool)
        n251 = Equal To 0?(x=w701) -> (x = 0?=w708:bool)
        n252 = case shown="False" w709 {
          tunnel: w703 -> [w724 w738]
          tunnel: w704 -> [w722 w731]
          tunnel: [w721 w730] -> w713
          tunnel: [w723 w739] -> w712
          tunnel: w711 -> [_ w736]
          tunnel: w708 -> [_ w737]
          frame False {
            n253 = Bundle By Name(cluster=w724, "Calc Speed.Calc 6"=FALSE ("Calc Speed.Calc 1")) -> (w723:T3)
            n254 = Insert Into Array(array=w722, index=0, new element="Find Header") -> (w721:string[])
          }
          frame True {
            n255 = To Double Precision Float(number=w736) -> (double precision float=w735:dbl[])
            n256 = case shown="False" w737 {
              tunnel: w738 -> [_ w744]
              tunnel: w735 -> [w740 w742]
              tunnel: [w740 w741] -> w734
              frame True {
              }
              frame False {
                n257 = Unbundle By Name(w744) -> ("Array 12"=w743:dbl[])
                n258 = Build Array (concatenate)(w743, w742) -> (w741:dbl[])
              }
            }
            n259 = Insert Into Array(array=w731, index=0, new element="Calc Speeds") -> (w730:string[])
            n260 = Bundle By Name(cluster=w738, "Array 12"=w734, "Calc Speed.Calc 6"=TRUE ("Calc Speed.Calc 1"), "PreRead Pts"=0) -> (w739:T3)
          }
        }
      }
      frame "Calc Speeds" {
        w751 = bool[] [TRUE, TRUE, TRUE, TRUE, TRUE, TRUE] ("Calc Speed")
        # "Global locked at No controller"
        n261 = Unbundle By Name(w757) -> ("Calc Speed"=w753:T2)
        n262 = Cluster To Array(cluster=w753) -> (array=w752:bool[])
        n263 = feedback #1(w751) -> (w749:bool[])
        n264 = feedback-in #1(w752) -> ()
        n265 = call "Speed Config Global.vi"() -> ("Speed Settings Out"=w748:T5, "Controller Out"=w746:bool, "Speed Enable Out"=w747:bool[])  [unwired: 13 in]
        n266 = Compound Arithmetic op=AND(invert w749, invert w751) -> (w750:bool[])
        n267 = case shown="False" w746 {
          tunnel: w757 -> [w758 w774]
          tunnel: w756 -> [w760 w773]
          tunnel: [w759 w772] -> w754
          tunnel: w750 -> [_ w771]
          tunnel: w749 -> [_ w770]
          tunnel: w748 -> [_ w769]
          tunnel: [w758 w763] -> w745
          tunnel: w747 -> [_ w766]
          frame True {
            # "Controller - leave FPGA crossing speed detection"
            n268 = Insert Into Array(array=w760, index=0, new element="Controller") -> (w759:string[])
          }
          frame False {
            # "No controller - Calculate speed here through FFT"
            n269 = for {
              tunnel: w771 -> [w780] mode=indexing
              tunnel: w770 -> [w782] mode=indexing
              shift-right: [w779] -> w763
              shift-left: w774 -> [w778]
              tunnel: w769 -> [w777]
              tunnel: w766 -> [w775] mode=indexing
              i -> [w781]
              n270 = flat-sequence {
                tunnel: [w854] -> w776
                frame #0 {
                  w854 = u32 5 ("milliseconds to wait")
                  n271 = Wait (ms)(milliseconds to wait=w854) -> ()  [unwired: 1 out]
                }
              }
              n272 = case shown="True" w775 {
                tunnel: w782 -> [_ w795]
                tunnel: w781 -> [w783 w794]
                tunnel: w780 -> [_ w793]
                tunnel: [w784 w792] -> w779
                tunnel: w778 -> [w785 w791]
                tunnel: w777 -> [_ w790]
                tunnel: w776 -> [_ w789]
                frame False {
                  n273 = Unbundle By Name(w785) -> ("Speeds"=w788:dbl[])
                  n274 = Replace Array Subset(array=w788, new element=0.0 ("Speeds.Speed 1"), index=w783) -> (w787:dbl[])
                  n275 = Bundle By Name(cluster=w785, "Speeds"=w787) -> (w784:T3)
                }
                frame True {
                  n276 = case shown="True" w795 {
                    tunnel: w794 -> [w798 w809]
                    tunnel: w793 -> [w799 _]
                    tunnel: w791 -> [w797 w815]
                    tunnel: [w796 w822] -> w792
                    tunnel: w790 -> [_ w807]
                    tunnel: w789 -> [_ _]
                    frame False {
                      n277 = case shown="True" w799 {
                        tunnel: w798 -> [_ w802]
                        tunnel: w797 -> [w800 w805]
                        tunnel: [w800 w806] -> w796
                        frame False {
                          # "No data on last read\n\nleave previous speed"
                        }
                        frame True {
                          # "Second time no data\nset speed to NaN"
                          n278 = Unbundle By Name(w805) -> ("Speeds"=w804:dbl[])
                          n279 = Replace Array Subset(array=w804, new element=nan ("Speeds.Speed 1"), index=w802) -> (w803:dbl[])
                          n280 = Bundle By Name(cluster=w805, "Speeds"=w803) -> (w806:T3)
                        }
                      }
                    }
                    frame True {
                      n281 = case shown="1" w809 {
                        tunnel: w815 -> [w828 w833 w838 w843 w848 w853]
                        tunnel: [w827 w832 w837 w842 w847 w852] -> w820
                        tunnel: [w826 w831 w836 w841 w846 w851] -> w823
                        tunnel: [w825 w830 w835 w840 w845 w850] -> w819
                        tunnel: [w824 w829 w834 w839 w844 w849] -> w808
                        frame 0, Default {
                          n282 = Unbundle By Name(w828) -> ("Speeds"=w826:dbl[], "Speeds 2"=w824:dbl[], "Array 1"=w827:dbl[], "Array 7"=w825:dbl[])
                        }
                        frame 1 {
                          n283 = Unbundle By Name(w833) -> ("Speeds"=w831:dbl[], "Speeds 2"=w829:dbl[], "Array 2"=w832:dbl[], "Array 8"=w830:dbl[])
                        }
                        frame 2 {
                          n284 = Unbundle By Name(w838) -> ("Speeds"=w836:dbl[], "Speeds 2"=w834:dbl[], "Array 3"=w837:dbl[], "Array 9"=w835:dbl[])
                        }
                        frame 3 {
                          n285 = Unbundle By Name(w843) -> ("Speeds"=w841:dbl[], "Speeds 2"=w839:dbl[], "Array 4"=w842:dbl[], "Array 10"=w840:dbl[])
                        }
                        frame 4 {
                          n286 = Unbundle By Name(w848) -> ("Speeds"=w846:dbl[], "Speeds 2"=w844:dbl[], "Array 5"=w847:dbl[], "Array 11"=w845:dbl[])
                        }
                        frame 5 {
                          n287 = Unbundle By Name(w853) -> ("Speeds"=w851:dbl[], "Speeds 2"=w849:dbl[], "Array 6"=w852:dbl[], "Array 12"=w850:dbl[])
                        }
                      }
                      n288 = call "Find Speed (Optimized).vi"("[x]"=w820, "Speed Settings"=w807, "index"=w809) -> ("Speed"=w818:dbl)  [unwired: 12 in]
                      n289 = call "Find Speed (Optimized).vi"("[x]"=w819, "Speed Settings"=w807) -> ("Speed"=w813:dbl)  [unwired: 13 in]
                      n290 = Add(x=w818, y=w813) -> (x+y=w812:dbl)
                      n291 = Index Array(array=w808, index=w809) -> (element=w811:dbl)
                      n292 = Add(x=w811, y=w812) -> (x+y=w810:dbl)
                      n293 = Multiply(x=w810, y=0.33333) -> (x*y=w816:dbl)
                      n294 = Replace Array Subset(array=w823, new element=w816, index=w809) -> (w821:dbl[])
                      n295 = Replace Array Subset(array=w808, new element=w813, index=w809) -> (w814:dbl[])
                      n296 = Bundle By Name(cluster=w815, "Speeds"=w821, "Speeds 2"=w814) -> (w822:T3)
                    }
                  }
                }
              }
            }
            n297 = Insert Into Array(array=w773, index=0, new element="Remove Buffer") -> (w772:string[])
            n298 = Unbundle By Name(w763) -> ("Speeds"=w765:dbl[])
            n299 = call "Tank Data Global.vi"("Speed"=w765, "Pump Data Mode"=Pump_Data_Mode."Write Speed") -> ()  [unwired: 13 in, 5 out]
          }
        }
      }
      frame "Remove Buffer" {
        n300 = flat-sequence {
          tunnel: [w869] -> w866
          tunnel: [w881] -> w865
          tunnel: [w868] -> w864
          tunnel: w860 -> [w881]
          tunnel: w859 -> [w869]
          tunnel: w858 -> [w868]
          tunnel: w866 -> [w896]
          tunnel: w865 -> [w895]
          tunnel: w864 -> [w885]
          tunnel: [w896] -> w863
          tunnel: [w884] -> w862
          tunnel: [w882] -> w861
          tunnel: [w908] -> w857
          tunnel: [w909] -> w855
          tunnel: [w905] -> w856
          tunnel: w863 -> [w906]
          tunnel: w862 -> [w909]
          tunnel: w861 -> [w908]
          frame #0 {
            # "Less than cycle time so that FIFO does not overflow"
            n301 = Unbundle By Name(w869) -> ("LoopStartTime"=w870:dbl)
            n302 = Get Date/Time In Seconds() -> (seconds since 1Jan1904=w879:timestamp)
            n303 = To Double Precision Float(number=w879) -> (double precision float=w878:dbl)
            n304 = Subtract(x=w878, y=w870) -> (x-y=w877:dbl)
            n305 = Multiply(x=w877, y=1000.0) -> (x*y=w875:dbl)
            n306 = To Unsigned Long Integer(number=w875) -> (unsigned 32bit integer=w873:u32)
            n307 = Subtract(x=u32 980, y=w873) -> (x-y=w872:u32)
            n308 = In Range and Coerce(upper limit=u32 300, x=w872, lower limit=u32 0) -> (coerced(x)=w880:u32)  [unwired: 1 out]
            n309 = Wait (ms)(milliseconds to wait=w880) -> ()  [unwired: 1 out]
          }
          frame #1 {
            n310 = while {
              shift-right: [w902] -> w893
              shift-left: w895 -> [w903]
              stop <- w897 stop-if-true
              n311 = xnode "Invoke Method"("FPGA VI Reference In"=w903, "Number of Elements"=u32 0) -> ("FPGA VI Reference Out"=w902:T1, "Elements Remaining"=w900:u32)  [unwired: 2 in, 2 out]
              n312 = Greater Or Equal?(x=w900, y=u32 1237 ("Number of Elements")) -> (x >= y?=w897:bool)
              n313 = Wait (ms)(milliseconds to wait=u32 2) -> ()  [unwired: 1 out]
            }
            n314 = xnode "Invoke Method"("FPGA VI Reference In"=w893, "Number of Elements"=u32 1238) -> ("FPGA VI Reference Out"=w882:T1, "Data"=w883:fxp<+/-,25,6>[])  [unwired: 2 in, 2 out]
            n315 = Delete From Array(array=w883) -> (deleted portion=w886:fxp<+/-,25,6>)  [unwired: 2 in, 1 out]
            n316 = Equal?(x=w886, y=fxp<+/-,25,6> -21.0) -> (x = y?=w888:bool)
            n317 = Select(t="First Pump 1", s=w888, f="Find Header") -> (s? t:f=w891:string)
            n318 = Insert Into Array(array=w885, index=0, new element=w891) -> (w884:string[])
          }
          frame #2 {
            n319 = Get Date/Time In Seconds() -> (seconds since 1Jan1904=w907:timestamp)
            n320 = To Double Precision Float(number=w907) -> (double precision float=w904:dbl)
            n321 = Bundle By Name(cluster=w906, "LoopStartTime"=w904) -> (w905:T3)
          }
        }
      }
      frame "Controller" {
        # "Global locked at No controller"
        n322 = xnode "Invoke Method"("FPGA VI Reference In"=w923, "Number of Elements"=u32 0) -> ("FPGA VI Reference Out"=w920:T1, "error out"=w919:errorcluster, "Elements Remaining"=w921:u32)  [unwired: 2 in, 1 out]
        n323 = call "Speed Config Global.vi"() -> ("Controller Out"=w915:bool)  [unwired: 13 in, 2 out]
        n324 = Wait (ms)(milliseconds to wait=u32 500) -> ()  [unwired: 1 out]
        n325 = Select(t="Controller", s=w915, f="Find Header") -> (s? t:f=w913:string)
        n326 = xnode "Invoke Method"("FPGA VI Reference In"=w920, "error in"=w919, "Number of Elements"=w921) -> ("FPGA VI Reference Out"=w918:T1)  [unwired: 1 in, 3 out]
        n327 = Insert Into Array(array=w910, index=0, new element=w913) -> (w911:string[])
      }
      frame "Header Error" {
        n328 = Wait (ms)(milliseconds to wait=u32 250) -> ()  [unwired: 1 out]
      }
    }
  }
